vi "Register Worker.vi"(8 "error in (no error)":errorcluster, 10 "Worker":refnum<class "Job Handler.lvclass">, 11 "Stub Worker Handler In":refnum<class "Stub Job Handler.lvclass">) -> (0 "error out":errorcluster, 3 "Stub Worker Handler Out":refnum<class "Stub Job Handler.lvclass">)   [LabVIEW 2020, in "Stub Job Handler.lvclass"]
uses:
  Stub Job Handler.lvclass
  Processes/People/Process Job/Job Handler.lvclass
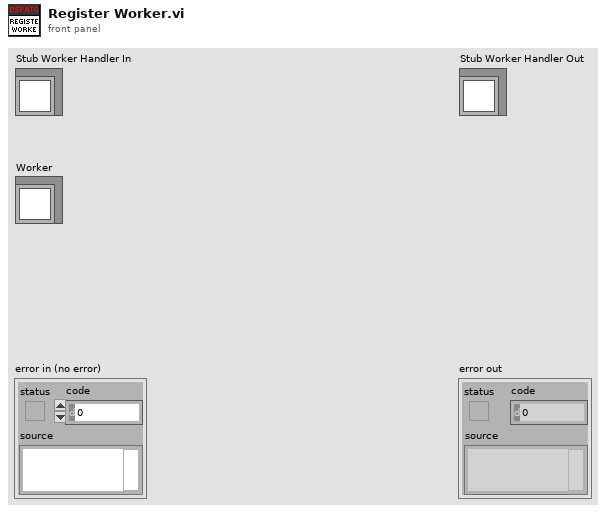
[diagram p1: front panel]
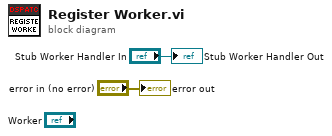
[diagram p0: block diagram]
diagram:
  "error out" <- "error in (no error)"
  "Stub Worker Handler Out" <- "Stub Worker Handler In"
